vi "Variant Array Interleave.vi"(8 "error in (no error)":errorcluster, 10 "Default Element Type":variant, 11 "Array of Variant Arrays":variant[](array[variant])) -> (0 "error out":errorcluster, 3 "N Dim Array out":variant)   [LabVIEW 2018, in "labview_json.lvlib"]
uses:
  labview_json.lvlib
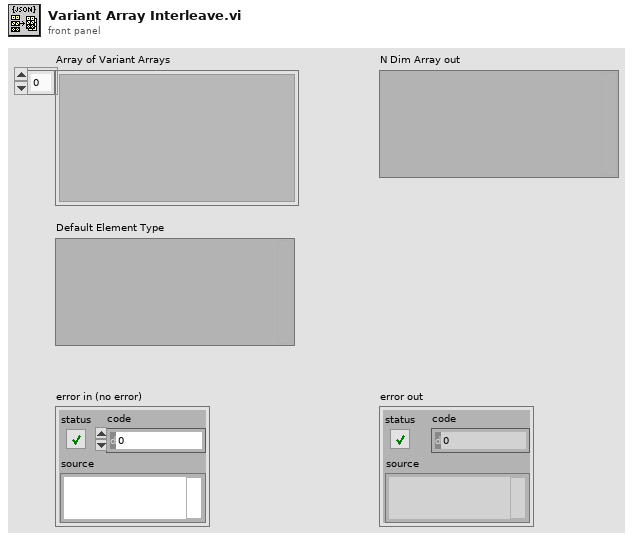
[diagram p1: front panel]
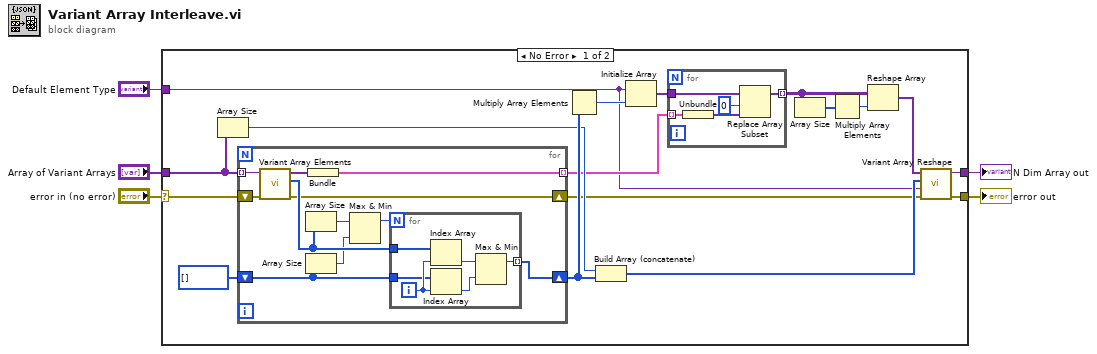
[diagram p0: block diagram]
diagram:
  n1 = case shown="No Error" "error in (no error)" {
    selector: "error in (no error)" -> [w22 w45]
    tunnel: "Array of Variant Arrays" -> [w19 _]
    tunnel: [w18 w45] -> w3
    tunnel: [w17 _] -> w2
    tunnel: "Default Element Type" -> [w6 _]
    frame No Error {
      n2 = Array Size(array=w19) -> (size(s)=w15:i32)
      n3 = for {
        tunnel: w19 -> [w37] mode=indexing
        shift-right: [w36] -> w16
        shift-left: i32[] [] -> [w35]
        shift-right: [w30] -> w7
        shift-left: w22 -> [w38]
        tunnel: [w28] -> w13 mode=indexing
        n4 = call "Variant Array Elements.vi"("error in (no error)"=w38, "N Dim Array"=w37) -> ("error out"=w30:errorcluster, "Sizes"=w34:i32[], "Elements"=w29:variant[])  [unwired: 6 in, 1 out]
        n5 = Array Size(array=w34) -> (size(s)=w33:i32)
        n6 = Array Size(array=w35) -> (size(s)=w32:i32)
        n7 = Bundle("Elements"=w29) -> (w28:cluster{"Elements":variant[]})  [unwired: 1 in]
        n8 = Max & Min(x=w33, y=w32) -> (max(x,y)=w31:i32)  [unwired: 1 out]
        n9 = for {
          N: w31 -> [_]
          tunnel: w34 -> [w44]
          tunnel: [w40] -> w36 mode=indexing
          tunnel: w35 -> [w39]
          i -> [w43]
          n10 = Index Array(array=w44, index=w43) -> (element=w42:i32)
          n11 = Index Array(array=w39, index=w43) -> (element=w41:i32)
          n12 = Max & Min(x=w42, y=w41) -> (max(x,y)=w40:i32)  [unwired: 1 out]
        }
      }
      n13 = Multiply Array Elements(1:w16) -> (0:w20:i32)
      n14 = Build Array (concatenate)(w15, w16) -> (w14:i32[])
      n15 = Initialize Array(w6, w20) -> (w12:variant[])
      n16 = for {
        tunnel: w13 -> [w26] mode=indexing
        tunnel: w12 -> [w27]
        tunnel: [w23] -> w11 mode=indexing
        n17 = Unbundle(w26) -> ("Elements"=w25:variant[])
        n18 = Replace Array Subset(array=w27, new element=w25, index=0) -> (w23:variant[])
      }
      n19 = Array Size(array=w11) -> (size(s)=w10:i32[])
      n20 = Multiply Array Elements(1:w10) -> (0:w9:i32)
      n21 = Reshape Array(w11, w9) -> (w8:variant[])
      n22 = call "Variant Array Reshape.vi"("error in (no error)"=w7, "Default Element Type"=w6, "Sizes"=w14, "Elements"=w8) -> ("error out"=w18:errorcluster, "N Dim Array"=w17:variant)  [unwired: 6 in]
    }
    frame Error {
    }
  }
  "N Dim Array out" <- w2
  "error out" <- w3
